vi "Strain gauge read.vi"() -> ()   [LabVIEW 2019]
uses:
  <vilib>/Analysis/NI_AALBase.lvlib
  SubVIs/Lake Shore 121/Lake Shore 121.lvlib
panel:
  in  "Current source":refnum<visa-resource-name>="COM7"
  out "Voltage 4a":cluster{"x":dbl, "y":dbl}[](graph)
  out "Voltage 3a":cluster{"x":dbl, "y":dbl}[](graph)
  out "Voltage 2a":cluster{"x":dbl, "y":dbl}[](graph)
  out "Voltage 1a":cluster{"x":dbl, "y":dbl}[](graph)
  out "Voltage 1b":cluster{"x":dbl, "y":dbl}[](graph)
  out "Voltage 2b":cluster{"x":dbl, "y":dbl}[](graph)
  out "Voltage 3b":cluster{"x":dbl, "y":dbl}[](graph)
  out "Voltage 4b":cluster{"x":dbl, "y":dbl}[](graph)
  out "Strain 4 error":dbl
  out "Strain 4":dbl
  out "Voltage 4 error":dbl
  out "Voltage 4":dbl format="%#_8g"
  out "Strain 3 error":dbl
  out "Strain 3":dbl
  out "Voltage 3 error":dbl
  out "Voltage 3":dbl format="%#_8g"
  out "Strain 2 error":dbl
  out "Strain 2":dbl
  out "Voltage 2 error":dbl
  out "Voltage 2":dbl format="%#_8g"
  out "Strain 1 error":dbl
  out "Strain 1":dbl
  out "Voltage 1 error":dbl
  out "Voltage 1":dbl format="%#_8g"
  in  "Voltage 4(BR)":refnum<visa-resource-name>="USB0::0x05E6::0x2100::1415939::INSTR"
  in  "Voltage 3(BL)":refnum<visa-resource-name>="USB0::0x05E6::0x2100::1269999::INSTR"
  in  "Voltage 2(TR)":refnum<visa-resource-name>="USB0::0x05E6::0x2100::1415930::INSTR"
  in  "Voltage 1(TL)":refnum<visa-resource-name>="USB0::0x05E6::0x2100::1310629::INSTR"
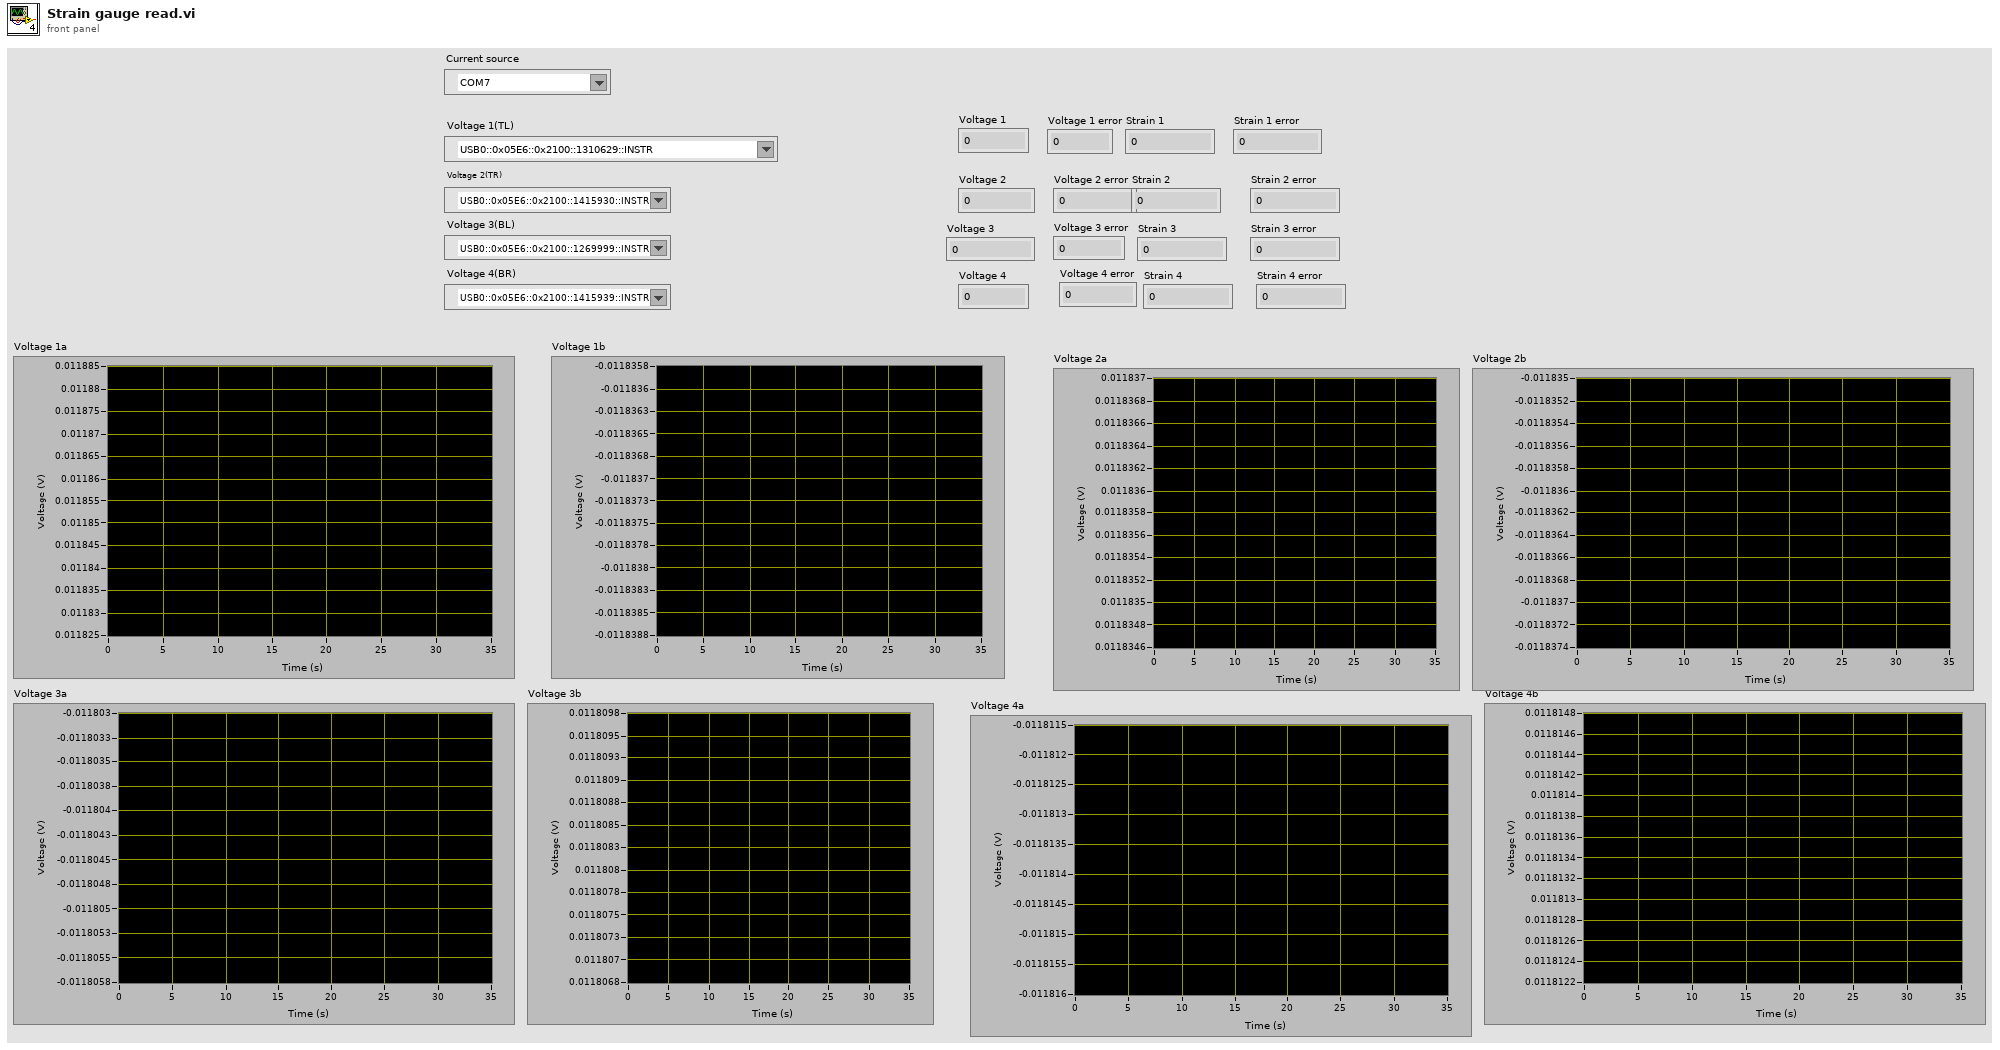
[diagram p1: front panel]
types:
  T1 = cluster{"Elapsed Time (s)":dbl, "Measurement":dbl}
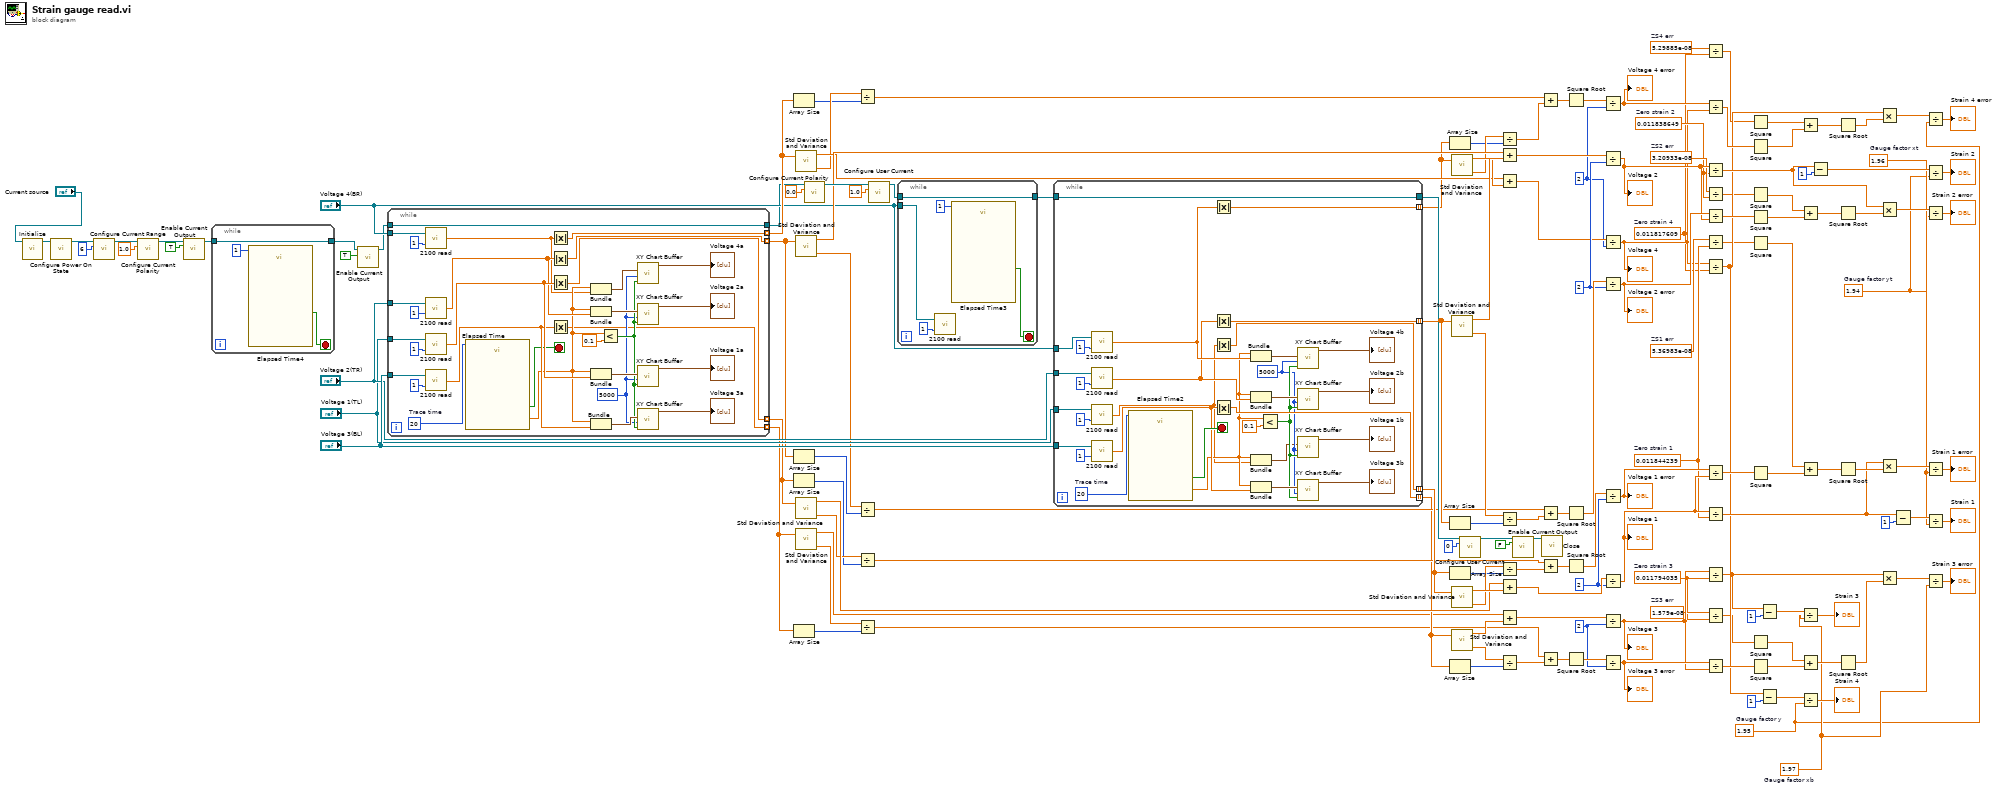
[diagram p0: block diagram]
diagram:
  w1 = 1.94  # Gauge factor yt
  w3 = 1.97  # Gauge factor xb
  w40 = 5.29885e-08  # ZS4 err
  w39 = 0.011817609  # Zero strain 4
  w46 = 2
  w68 = 1.579e-08  # ZS3 err
  w67 = 0.011794035  # Zero strain 3
  w74 = 2
  w94 = 3.20933e-08  # ZS2 err
  w93 = 0.011838649  # Zero strain 2
  w100 = 2
  w116 = 5.36983e-08  # ZS1 err
  w2 = 1.95  # Gauge factor y
  w12 = 1.96  # Gauge factor xt
  w115 = 0.011844239  # Zero strain 1
  w122 = 2
  n1 = call "Initialize.vi"("VISA resource name"="Current source") -> ("VISA resource name out"=w150:refnum<visa-resource-name>)  [unwired: 9 in, 1 out]
  n2 = call "Configure Power On State.vi"("VISA resource name"=w150) -> ("VISA resource name out"=w148:refnum<visa-resource-name>)  [unwired: 13 in, 1 out]
  n3 = call "Configure Current Range.vi"("Output Current Range (0:100 nA)"=6, "VISA resource name"=w148) -> ("VISA resource name out"=w14:refnum<visa-resource-name>)  [unwired: 8 in, 1 out]
  n4 = call "Configure Current Polarity.vi"("VISA resource name"=w14, "Polarity (0:Positive)"=1.0) -> ("VISA resource name out"=w15:refnum<visa-resource-name>)  [unwired: 12 in, 1 out]
  n5 = call "Enable Current Output.vi"("VISA resource name"=w15, "Enable Current Output (F: Disable)"=TRUE) -> ("VISA resource name out"=w18:refnum<visa-resource-name>)  [unwired: 12 in, 1 out]
  n6 = while {
    tunnel: [w154] -> w6
    tunnel: w18 -> [w154]
    stop <- w153 stop-if-true
    n7 = call "Elapsed Time4"("Time Target (s)"=1) -> ("Time has Elapsed"=w153:bool)  [unwired: 11 in, 7 out]
  }
  n8 = call "Enable Current Output.vi"("VISA resource name"=w6, "Enable Current Output (F: Disable)"=TRUE) -> ("VISA resource name out"=w5:refnum<visa-resource-name>)  [unwired: 12 in, 1 out]
  n9 = while {
    tunnel: [w157] -> w10 mode=indexing
    tunnel: [w155] -> w8 mode=indexing
    tunnel: [w158] -> w30 mode=indexing
    tunnel: w5 -> [w164]
    tunnel: [w164] -> w11
    tunnel: "Voltage 3(BL)" -> [w160]
    tunnel: "Voltage 2(TR)" -> [w161]
    tunnel: "Voltage 1(TL)" -> [w162]
    tunnel: "Voltage 4(BR)" -> [w163]
    tunnel: [w156] -> w9 mode=indexing
    stop <- w159 stop-if-true
    w168 = 5000
    w181 = 20  # Trace time
    n10 = call "2100 read.vi"("Gain"=1, "VISA resource name"=w163) -> ("Measurement"=w165:dbl)
    n11 = call "2100 read.vi"("Gain"=1, "VISA resource name"=w161) -> ("Measurement"=w175:dbl)
    n12 = call "2100 read.vi"("Gain"=1, "VISA resource name"=w162) -> ("Measurement"=w179:dbl)
    n13 = call "2100 read.vi"("Gain"=1, "VISA resource name"=w160) -> ("Measurement"=w171:dbl)
    n14 = call "Elapsed Time"("Time Target (s)"=w181) -> ("Elapsed Time (s)"=w166:dbl, "Time has Elapsed"=w159:bool)  [unwired: 11 in, 6 out]
    n15 = Absolute Value(x=w165) -> (abs(x)=w158:dbl)
    n16 = Absolute Value(x=w175) -> (abs(x)=w155:dbl)
    n17 = Absolute Value(x=w179) -> (abs(x)=w157:dbl)
    n18 = Absolute Value(x=w171) -> (abs(x)=w156:dbl)
    n19 = Bundle "Bundle"("Elapsed Time (s)"=w166, "Measurement"=w165) -> (w167:T1)  [unwired: 1 in]
    n20 = Bundle "Bundle"("Elapsed Time (s)"=w166, "Measurement"=w175) -> (w176:T1)  [unwired: 1 in]
    n21 = Bundle "Bundle"("Elapsed Time (s)"=w166, "Measurement"=w179) -> (w178:T1)  [unwired: 1 in]
    n22 = Bundle "Bundle"("Elapsed Time (s)"=w166, "Measurement"=w171) -> (w172:T1)  [unwired: 1 in]
    n23 = Less?(x=w166, y=0.1) -> (x < y?=w169:bool)
    n24 = call "XY Chart Buffer.vi"("clear first (no:F)"=w169, "chart length (points)"=w168, "new point"=w167) -> ("XY chart data"=→"Voltage 4a":cluster{"x":dbl, "y":dbl}[])  [unwired: 8 in]
    n25 = call "XY Chart Buffer.vi"("clear first (no:F)"=w169, "chart length (points)"=w168, "new point"=w176) -> ("XY chart data"=→"Voltage 2a":cluster{"x":dbl, "y":dbl}[])  [unwired: 8 in]
    n26 = call "XY Chart Buffer.vi"("clear first (no:F)"=w169, "chart length (points)"=w168, "new point"=w178) -> ("XY chart data"=→"Voltage 1a":cluster{"x":dbl, "y":dbl}[])  [unwired: 8 in]
    n27 = call "XY Chart Buffer.vi"("clear first (no:F)"=w169, "chart length (points)"=w168, "new point"=w172) -> ("XY chart data"=→"Voltage 3a":cluster{"x":dbl, "y":dbl}[])  [unwired: 8 in]
  }
  n28 = Array Size(array=w30) -> (size(s)=w28:i32)
  n29 = Array Size(array=w8) -> (size(s)=w84:i32)
  n30 = Array Size(array=w10) -> (size(s)=w125:i32)
  n31 = Array Size(array=w9) -> (size(s)=w55:i32)
  n32 = call <vilib>:"Std Deviation and Variance.vi"("X"=w30) -> ("mean"=w31:dbl, "variance"=w29:dbl)  [unwired: 1 in, 1 out]
  n33 = call <vilib>:"Std Deviation and Variance.vi"("X"=w8) -> ("mean"=w57:dbl, "variance"=w83:dbl)  [unwired: 1 in, 1 out]
  n34 = call <vilib>:"Std Deviation and Variance.vi"("X"=w10) -> ("mean"=w132:dbl, "variance"=w126:dbl)  [unwired: 1 in, 1 out]
  n35 = call <vilib>:"Std Deviation and Variance.vi"("X"=w9) -> ("mean"=w56:dbl, "variance"=w58:dbl)  [unwired: 1 in, 1 out]
  n36 = call "Configure Current Polarity.vi"("VISA resource name"=w11, "Polarity (0:Positive)"=0.0) -> ("VISA resource name out"=w142:refnum<visa-resource-name>)  [unwired: 12 in, 1 out]
  n37 = Divide(x=w29, y=w28) -> (x/y=w27:dbl)
  n38 = Divide(x=w83, y=w84) -> (x/y=w82:dbl)
  n39 = Divide(x=w126, y=w125) -> (x/y=w124:dbl)
  n40 = Divide(x=w58, y=w55) -> (x/y=w54:dbl)
  n41 = call "Configure User Current.vi"("VISA resource name"=w142, "User Current (100E-9)"=1.0) -> ("VISA resource name out"=w136:refnum<visa-resource-name>)  [unwired: 12 in, 1 out]
  n42 = while {
    tunnel: [w190] -> w135
    tunnel: w136 -> [w190]
    tunnel: "Voltage 4(BR)" -> [w187]
    stop <- w189 stop-if-true
    n43 = call "2100 read.vi"("Gain"=1, "VISA resource name"=w187) -> ()  [unwired: 1 out]
    n44 = call "Elapsed Time3"("Time Target (s)"=1) -> ("Time has Elapsed"=w189:bool)  [unwired: 11 in, 7 out]
  }
  n45 = while {
    tunnel: [w214] -> w59 mode=indexing
    tunnel: [w212] -> w134 mode=indexing
    tunnel: [w215] -> w85 mode=indexing
    tunnel: [w213] -> w16 mode=indexing
    tunnel: [w211] -> w146
    tunnel: w135 -> [w211]
    tunnel: "Voltage 1(TL)" -> [w210]
    tunnel: "Voltage 2(TR)" -> [w209]
    tunnel: "Voltage 3(BL)" -> [w208]
    tunnel: "Voltage 4(BR)" -> [w207]
    stop <- w217 stop-if-true
    w194 = 5000
    w216 = 20  # Trace time
    n46 = call "2100 read.vi"("Gain"=1, "VISA resource name"=w207) -> ("Measurement"=w205:dbl)
    n47 = call "2100 read.vi"("Gain"=1, "VISA resource name"=w209) -> ("Measurement"=w197:dbl)
    n48 = call "2100 read.vi"("Gain"=1, "VISA resource name"=w210) -> ("Measurement"=w191:dbl)
    n49 = call "2100 read.vi"("Gain"=1, "VISA resource name"=w208) -> ("Measurement"=w201:dbl)
    n50 = call "Elapsed Time2"("Time Target (s)"=w216) -> ("Elapsed Time (s)"=w192:dbl, "Time has Elapsed"=w217:bool)  [unwired: 11 in, 6 out]
    n51 = Absolute Value(x=w205) -> (abs(x)=w213:dbl)
    n52 = Absolute Value(x=w197) -> (abs(x)=w215:dbl)
    n53 = Absolute Value(x=w191) -> (abs(x)=w212:dbl)
    n54 = Absolute Value(x=w201) -> (abs(x)=w214:dbl)
    n55 = Bundle "Bundle"("Elapsed Time (s)"=w192, "Measurement"=w205) -> (w204:T1)  [unwired: 1 in]
    n56 = Bundle "Bundle"("Elapsed Time (s)"=w192, "Measurement"=w197) -> (w198:T1)  [unwired: 1 in]
    n57 = Bundle "Bundle"("Elapsed Time (s)"=w192, "Measurement"=w191) -> (w193:T1)  [unwired: 1 in]
    n58 = Bundle "Bundle"("Elapsed Time (s)"=w192, "Measurement"=w201) -> (w202:T1)  [unwired: 1 in]
    n59 = Less?(x=w192, y=0.1) -> (x < y?=w195:bool)
    n60 = call "XY Chart Buffer.vi"("clear first (no:F)"=w195, "chart length (points)"=w194, "new point"=w204) -> ("XY chart data"=→"Voltage 4b":cluster{"x":dbl, "y":dbl}[])  [unwired: 8 in]
    n61 = call "XY Chart Buffer.vi"("clear first (no:F)"=w195, "chart length (points)"=w194, "new point"=w198) -> ("XY chart data"=→"Voltage 2b":cluster{"x":dbl, "y":dbl}[])  [unwired: 8 in]
    n62 = call "XY Chart Buffer.vi"("clear first (no:F)"=w195, "chart length (points)"=w194, "new point"=w193) -> ("XY chart data"=→"Voltage 1b":cluster{"x":dbl, "y":dbl}[])  [unwired: 8 in]
    n63 = call "XY Chart Buffer.vi"("clear first (no:F)"=w195, "chart length (points)"=w194, "new point"=w202) -> ("XY chart data"=→"Voltage 3b":cluster{"x":dbl, "y":dbl}[])  [unwired: 8 in]
  }
  n64 = Array Size(array=w16) -> (size(s)=w50:i32)
  n65 = Array Size(array=w85) -> (size(s)=w104:i32)
  n66 = Array Size(array=w134) -> (size(s)=w129:i32)
  n67 = Array Size(array=w59) -> (size(s)=w78:i32)
  n68 = call <vilib>:"Std Deviation and Variance.vi"("X"=w16) -> ("mean"=w53:dbl, "variance"=w51:dbl)  [unwired: 1 in, 1 out]
  n69 = call <vilib>:"Std Deviation and Variance.vi"("X"=w85) -> ("mean"=w107:dbl, "variance"=w105:dbl)  [unwired: 1 in, 1 out]
  n70 = call <vilib>:"Std Deviation and Variance.vi"("X"=w134) -> ("mean"=w133:dbl, "variance"=w130:dbl)  [unwired: 1 in, 1 out]
  n71 = call <vilib>:"Std Deviation and Variance.vi"("X"=w59) -> ("mean"=w81:dbl, "variance"=w79:dbl)  [unwired: 1 in, 1 out]
  n72 = call "Configure User Current.vi"("VISA resource name"=w146, "User Current (100E-9)"=0) -> ("VISA resource name out"=w144:refnum<visa-resource-name>)  [unwired: 12 in, 1 out]
  n73 = Divide(x=w51, y=w50) -> (x/y=w49:dbl)
  n74 = Add(x=w57, y=w107) -> (x+y=w106:dbl)
  n75 = Add(x=w31, y=w53) -> (x+y=w52:dbl)
  n76 = Divide(x=w105, y=w104) -> (x/y=w103:dbl)
  n77 = Divide(x=w130, y=w129) -> (x/y=w128:dbl)
  n78 = Add(x=w132, y=w133) -> (x+y=w131:dbl)
  n79 = Add(x=w56, y=w81) -> (x+y=w80:dbl)
  n80 = Divide(x=w79, y=w78) -> (x/y=w77:dbl)
  n81 = call "Enable Current Output.vi"("VISA resource name"=w144, "Enable Current Output (F: Disable)"=FALSE) -> ("VISA resource name out"=w143:refnum<visa-resource-name>)  [unwired: 12 in, 1 out]
  n82 = Add(x=w27, y=w49) -> (x+y=w48:dbl)
  n83 = Add(x=w82, y=w103) -> (x+y=w102:dbl)
  n84 = Add(x=w124, y=w128) -> (x+y=w127:dbl)
  n85 = Add(x=w54, y=w77) -> (x+y=w76:dbl)
  n86 = call "Close.vi"("VISA resource name"=w143) -> ()  [unwired: 10 in, 1 out]
  n87 = Square Root(x=w48) -> (sqrt(x)=w47:dbl)
  n88 = Square Root(x=w102) -> (sqrt(x)=w101:dbl)
  n89 = Square Root(x=w127) -> (sqrt(x)=w123:dbl)
  n90 = Square Root(x=w76) -> (sqrt(x)=w75:dbl)
  n91 = Divide(x=w47, y=w46) -> (x/y=w44:dbl)
  "Voltage 4 error" <- w44
  n92 = Divide(x=w106, y=w100) -> (x/y=w97:dbl)
  "Voltage 2" <- w97
  n93 = Divide(x=w52, y=w46) -> (x/y=w43:dbl)
  "Voltage 4" <- w43
  n94 = Divide(x=w101, y=w100) -> (x/y=w98:dbl)
  "Voltage 2 error" <- w98
  n95 = Divide(x=w123, y=w122) -> (x/y=w120:dbl)
  "Voltage 1 error" <- w120
  n96 = Divide(x=w131, y=w122) -> (x/y=w119:dbl)
  "Voltage 1" <- w119
  n97 = Divide(x=w80, y=w74) -> (x/y=w71:dbl)
  "Voltage 3" <- w71
  n98 = Divide(x=w75, y=w74) -> (x/y=w72:dbl)
  "Voltage 3 error" <- w72
  n99 = Divide(x=w40, y=w39) -> (x/y=w20:dbl)
  n100 = Divide(x=w44, y=w43) -> (x/y=w42:dbl)
  n101 = Divide(x=w97, y=w93) -> (x/y=w90:dbl)
  n102 = Divide(x=w94, y=w93) -> (x/y=w23:dbl)
  n103 = Divide(x=w98, y=w97) -> (x/y=w96:dbl)
  n104 = Divide(x=w116, y=w115) -> (x/y=w22:dbl)
  n105 = Divide(x=w43, y=w39) -> (x/y=w36:dbl)
  n106 = Divide(x=w120, y=w119) -> (x/y=w118:dbl)
  n107 = Divide(x=w119, y=w115) -> (x/y=w112:dbl)
  n108 = Divide(x=w71, y=w67) -> (x/y=w64:dbl)
  n109 = Divide(x=w68, y=w67) -> (x/y=w26:dbl)
  n110 = Divide(x=w72, y=w71) -> (x/y=w70:dbl)
  n111 = Square(x=w20) -> (x^2=w19:dbl)
  n112 = Square(x=w42) -> (x^2=w41:dbl)
  n113 = Square(x=w23) -> (x^2=w24:dbl)
  n114 = Square(x=w96) -> (x^2=w95:dbl)
  n115 = Square(x=w22) -> (x^2=w21:dbl)
  n116 = Square(x=w118) -> (x^2=w117:dbl)
  n117 = Square(x=w26) -> (x^2=w25:dbl)
  n118 = Square(x=w70) -> (x^2=w69:dbl)
  n119 = Subtract(x=w64, y=1) -> (x-y=w61:dbl)
  n120 = Subtract(x=w36, y=1) -> (x-y=w33:dbl)
  n121 = Add(x=w19, y=w41) -> (x+y=w38:dbl)
  n122 = Add(x=w24, y=w95) -> (x+y=w92:dbl)
  n123 = Add(x=w21, y=w117) -> (x+y=w114:dbl)
  n124 = Divide(x=w61, y=w3) -> (x/y=→"Strain 3":dbl)
  n125 = Add(x=w25, y=w69) -> (x+y=w66:dbl)
  n126 = Divide(x=w33, y=w2) -> (x/y=→"Strain 4":dbl)
  n127 = Subtract(x=w90, y=1) -> (x-y=w87:dbl)
  n128 = Square Root(x=w38) -> (sqrt(x)=w37:dbl)
  n129 = Square Root(x=w92) -> (sqrt(x)=w91:dbl)
  n130 = Square Root(x=w114) -> (sqrt(x)=w113:dbl)
  n131 = Square Root(x=w66) -> (sqrt(x)=w65:dbl)
  n132 = Multiply(x=w36, y=w37) -> (x*y=w35:dbl)
  n133 = Multiply(x=w90, y=w91) -> (x*y=w89:dbl)
  n134 = Multiply(x=w112, y=w113) -> (x*y=w111:dbl)
  n135 = Multiply(x=w64, y=w65) -> (x*y=w63:dbl)
  n136 = Subtract(x=w112, y=1) -> (x-y=w109:dbl)
  n137 = Divide(x=w35, y=w2) -> (x/y=→"Strain 4 error":dbl)
  n138 = Divide(x=w87, y=w1) -> (x/y=→"Strain 2":dbl)
  n139 = Divide(x=w89, y=w1) -> (x/y=→"Strain 2 error":dbl)
  n140 = Divide(x=w111, y=w12) -> (x/y=→"Strain 1 error":dbl)
  n141 = Divide(x=w109, y=w12) -> (x/y=→"Strain 1":dbl)
  n142 = Divide(x=w63, y=w3) -> (x/y=→"Strain 3 error":dbl)
